vi "Configure External Signal Generator.vi"(0 "VISA resource name":refnum<visa-resource-name>, 1 "Gpib Address (19)":i32=19, 2 "Type (3)":i32=3, 5 "Frequency Setting Command (FR %f% HZ)":string="FR %f% HZ", 7 "Power Level Setting Command (AP %P% DM)":string="AP %P% DM", 9 "Preset Command (\"\")":string, 11 "error in (no error)":errorcluster, 12 "RF Power On Command (R3)":string="R3", 13 "Waiting Time (0.10)":dbl=0.1 format="%.2f") -> (4 "VISA resource name out":refnum<visa-resource-name>, 15 "error out":errorcluster)   [LabVIEW 2020, in "Agilent ENA Series.lvlib"]
doc: "Configures the external signal generator.\n\n<b>Note:</b>\nThis VI is not supported by the E5063A, E5080A and E5080B."
uses:
  <instrlib>/Agilent ENA Series/Agilent ENA Series.lvlib
panel:
  # "Note:\nThis VI is not supported by the E5063A, E5080A and E5080B."
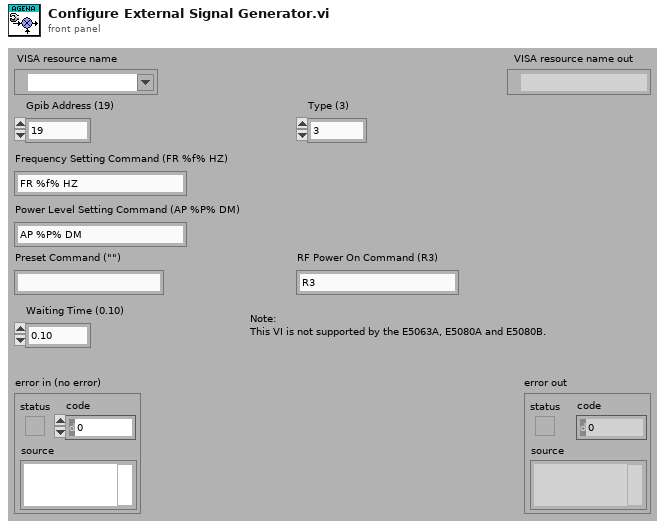
[diagram p1: front panel]
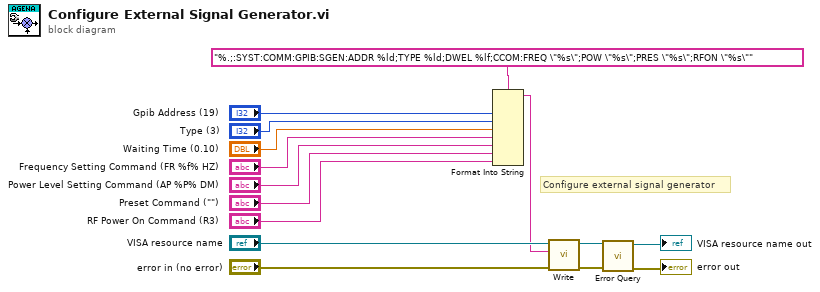
[diagram p0: block diagram]
diagram:
  # "Configure external signal generator"
  n1 = Format Into String(format string="%.;:SYST:COMM:GPIB:SGEN:ADDR %ld;TYPE %ld;DWEL %lf;CCOM:FREQ \"%s\";POW \"%s\";PRES \"%s\";RFON \"%s\"", "Gpib Address (19)", "Type (3)", "Waiting Time (0.10)", "Frequency Setting Command (FR %f% HZ)", "Power Level Setting Command (AP %P% DM)", "Preset Command (\"\")", "RF Power On Command (R3)") -> (resulting string=w5:string)  [unwired: 2 in, 1 out]
  n2 = call <instrlib>:"Write.vi"("error in (no error)"="error in (no error)", "String ()"=w5, "VISA resource name"="VISA resource name") -> ("error out"=w3:errorcluster, "VISA resource name out"=w4:refnum<visa-resource-name>)  [unwired: 6 in, 1 out]
  n3 = call <instrlib>:"Error Query.vi"("error in (no error)"=w3, "VISA resource name"=w4) -> ("error out"=→"error out":errorcluster, "VISA resource name out"=→"VISA resource name out":refnum<visa-resource-name>)  [unwired: 6 in, 2 out]
